vi "Test Data 2.vi"(8 "error in (no error)":errorcluster, 11 "Instrument.Lockin in":refnum<class "Instrument.Lockin.lvclass">) -> (0 "error out":errorcluster, 3 "Instrument.Lockin out":refnum<class "Instrument.Lockin.lvclass">)   [LabVIEW 2019]
uses:
  <vilib>/addons/_JKI Toolkits/Caraya/classes/Test/Test.lvclass
  src/Instrument.Lockin/Instrument.Lockin.lvclass
  src/Lockin.DAQ/Typedefs/AO_Channel-Numeric.ctl
  src/Lockin.DAQ/Lockin.DAQ.lvclass
  <vilib>/addons/_JKI Toolkits/Caraya/classes/Assert/Assert.lvclass
  <vilib>/addons/_JKI Toolkits/Caraya/classes/Assert/Assert Not Error.vi
  <vilib>/addons/_JKI Toolkits/Caraya/classes/Assert/Assert False.vi
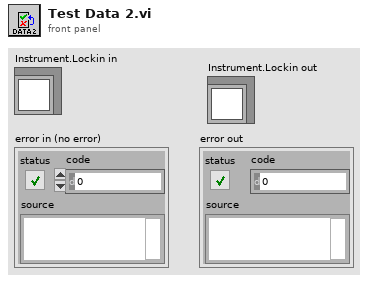
[diagram p1: front panel]
types:
  T1 = typedef "Lockin.DAQ.lvclass/AO_Channel-Numeric.ctl" = i32
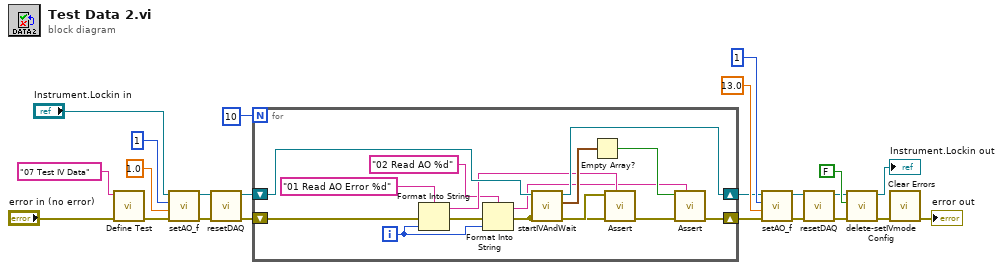
[diagram p0: block diagram]
diagram:
  n1 = call <vilib>:"Define Test.vi"("error in (no error)"="error in (no error)", "Label (VI Title)"="07 Test IV Data") -> ("error out"=w20:errorcluster)  [unwired: 9 in]
  n2 = call "setAO_f.vi"("error in (no error)"=w20, "Frequency (Hz)"=1.0, "AO Channel"=T1 1, "Instrument.Lockin in"="Instrument.Lockin in") -> ("error out"=w12:errorcluster, "Instrument.Lockin out"=w11:refnum<class "Instrument.Lockin.lvclass">)  [unwired: 6 in]
  n3 = call "resetDAQ.vi"("error in (no error)"=w12, "Instrument.Lockin in"=w11) -> ("error out"=w10:errorcluster, "Instrument.Lockin out"=w9:refnum<class "Instrument.Lockin.lvclass">)  [unwired: 8 in]
  n4 = for {
    N: 10 -> [_]
    shift-right: [w35] -> w14
    shift-left: w10 -> [w27]
    shift-right: [w34] -> w13
    shift-left: w9 -> [w33]
    i -> [w28]
    n5 = Format Into String(format string="01 Read AO Error %d" ("Label"), error in=w27, w28) -> (resulting string=w31:string, error out=w26:errorcluster)  [unwired: 1 in]
    n6 = Format Into String(format string="02 Read AO %d" ("Label"), error in=w26, w28) -> (resulting string=w29:string, error out=w24:errorcluster)  [unwired: 1 in]
    n7 = call "startIVAndWait.vi"("error in (no error)"=w24, "Instrument.Lockin in"=w33) -> ("error out"=w25:errorcluster, "AI Waveform"=w36:waveform(dbl)[], "Instrument.Lockin out"=w34:refnum<class "Instrument.Lockin.lvclass">)  [unwired: 7 in]
    n8 = Empty Array?(array=w36) -> (empty?=w38:bool)
    n9 = call-poly <vilib>:"Assert.vi"("Label"=w31, "error in (no error)"=w24, "Not Error?"=w25) -> ("error out"=w37:errorcluster)  [unwired: 8 in]
    n10 = call-poly <vilib>:"Assert.vi"("Label"=w29, "error in (no error)"=w37, "False?"=w38) -> ("error out"=w35:errorcluster)  [unwired: 8 in]
  }
  n11 = call "setAO_f.vi"("error in (no error)"=w14, "Frequency (Hz)"=13.0, "AO Channel"=T1 1, "Instrument.Lockin in"=w13) -> ("error out"=w6:errorcluster, "Instrument.Lockin out"=w5:refnum<class "Instrument.Lockin.lvclass">)  [unwired: 6 in]
  n12 = call "resetDAQ.vi"("error in (no error)"=w6, "Instrument.Lockin in"=w5) -> ("error out"=w3:errorcluster, "Instrument.Lockin out"=w4:refnum<class "Instrument.Lockin.lvclass">)  [unwired: 8 in]
  n13 = call "delete-setIVmodeConfig.vi"("error in (no error)"=w3, "IV mode"=FALSE, "Instrument.Lockin in"=w4) -> ("error out"=w2:errorcluster, "Instrument.Lockin out"=→"Instrument.Lockin out":refnum<class "Instrument.Lockin.lvclass">)  [unwired: 7 in]
  n14 = call <vilib>:"Clear Errors.vi"("error in (no error)"=w2) -> ("error out"=→"error out":errorcluster)  [unwired: 5 in, 1 out]
